vi "Images - Delete all png images.vi"(8 "Error In":errorcluster, 11 "Folder In":path) -> (0 "Error Out":errorcluster)   [LabVIEW 2011]
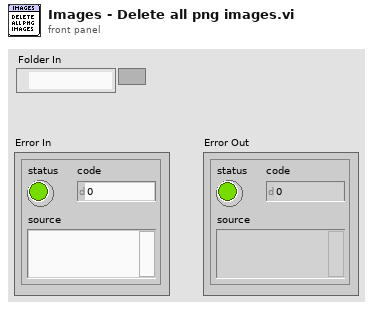
[diagram p1: front panel]
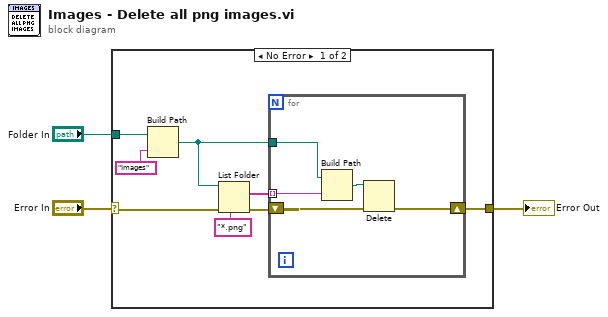
[diagram p0: block diagram]
diagram:
  n1 = case shown="No Error" "Error In" {
    selector: "Error In" -> [w10 w17]
    tunnel: "Folder In" -> [w6 _]
    tunnel: [w11 w17] -> w1
    frame No Error {
      n2 = Build Path(base path=w6, name or relative path="Images") -> (appended path=w5:path)
      n3 = List Folder(path=w5, pattern="*.png", error in=w10) -> (filenames=w8:string[], error out=w7:errorcluster)  [unwired: 1 in, 2 out]
      n4 = for {
        shift-right: [w16] -> w11
        shift-left: w7 -> [w12]
        tunnel: w8 -> [w13] mode=indexing
        tunnel: w5 -> [w15]
        n5 = Build Path(base path=w15, name or relative path=w13) -> (appended path=w14:path)
        n6 = Delete(path (use dialog)=w14, error in=w12) -> (error out=w16:errorcluster)  [unwired: 3 in, 2 out]
      }
    }
    frame Error {
    }
  }
  "Error Out" <- w1
